vi "Filter Control Terms.vi"(11 "Terms[]":refnum<vi>[](array[refnum])) -> (3 "Terms[] out":refnum<vi>[](array[refnum]))   [LabVIEW 2017, in "CSM-Helper.lvclass"]
uses:
  CSM-Helper.lvclass
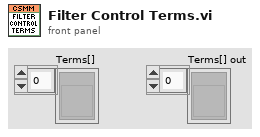
[diagram p1: front panel]
types:
  T1 = typedef "LVPositionTypeDef.ctl" = cluster{"Left":i32, "Top":i32}
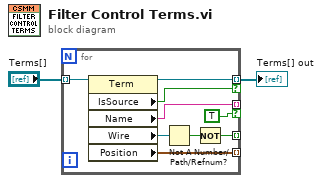
[diagram p0: block diagram]
diagram:
  n1 = for {
    tunnel: "Terms[]" -> [w11] mode=indexing
    tunnel: [w10] -> _ mode=indexing if=TRUE
    tunnel: [w7] -> _ mode=indexing
    tunnel: [w5] -> _ mode=indexing
    tunnel: [w4] -> w1 mode=indexing if=w9
    n2 = property class="Term"(reference=w11) -> (reference out=w4:refnum<vi>, "IsSource"=w9:bool, "Name"=w10:string, "Wire"=w8:refnum<vi>, "Position"=w5:T1)  [unwired: 1 in, 1 out]
    n3 = Not A Number/Path/Refnum?(number/path/refnum=w8) -> (NaN/Path/Refnum?=w3:bool)
    n4 = Not(x=w3) -> (.not. x?=w7:bool)
  }
  "Terms[] out" <- w1
